vi "Get Tolerance Value.vi"(10 "Tol sel":T2, 11 "# Bands":T1 min=3 max=6 step=1) -> (3 "Numeric":dbl)   [LabVIEW 2018]
uses:
  Tolerance--enum.ctl
  Number of Bands--number.ctl
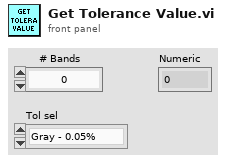
[diagram p1: front panel]
types:
  T1 = typedef "Number of Bands--number.ctl" = u8
  T2 = typedef "Tolerance--enum.ctl" = enum16{"Gray - 0.05%", "Violet - 0.1%", "Blue - 0.25%", "Green - 0.5%", "Brown - 1%", "Red - 2%", "Gold - 5%", "Silver - 10%", "None - 20%"}
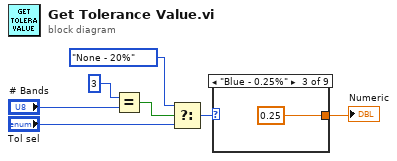
[diagram p0: block diagram]
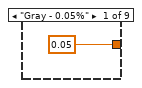
[diagram p2: hidden frame]
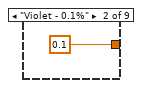
[diagram p3: hidden frame]
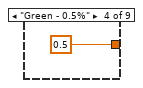
[diagram p4: hidden frame]
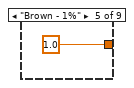
[diagram p5: hidden frame]
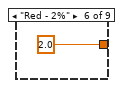
[diagram p6: hidden frame]
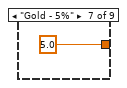
[diagram p7: hidden frame]
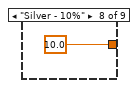
[diagram p8: hidden frame]
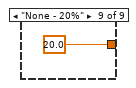
[diagram p9: hidden frame]
diagram:
  n1 = Equal?(x=T1 3 ("y"), y="# Bands") -> (x = y?=w2:bool)
  n2 = Select(t=Tolerance--enum."None - 20%", s=w2, f="Tol sel") -> (s? t:f=w7:T2)
  n3 = case shown="\"Blue - 0.25%\"" w7 {
    tunnel: [0.05 0.1 0.25 0.5 1.0 2.0 5.0 10.0 20.0] -> w1
    frame "Gray - 0.05%" {
    }
    frame "Violet - 0.1%" {
    }
    frame "Blue - 0.25%" {
    }
    frame "Green - 0.5%" {
    }
    frame "Brown - 1%" {
    }
    frame "Red - 2%" {
    }
    frame "Gold - 5%" {
    }
    frame "Silver - 10%" {
    }
    frame "None - 20%" {
    }
  }
  "Numeric" <- w1
